vi "Write Expected Image.vi"(8 "error in (no error)":errorcluster, 10 "image data":T1, 11 "Image Assertion in":refnum<class "Image Assertion.lvclass">) -> (0 "error out":errorcluster, 3 "Image Assertion out":refnum<class "Image Assertion.lvclass">)   [LabVIEW 2020, in "MacroAssert.lvlib" / "Image Assertion.lvclass"]
uses:
  Image Assertion.lvclass
  Image Assertion.lvclass/Image Assertion.ctl
  <vilib>/picture/picture.llb/imagedata.ctl
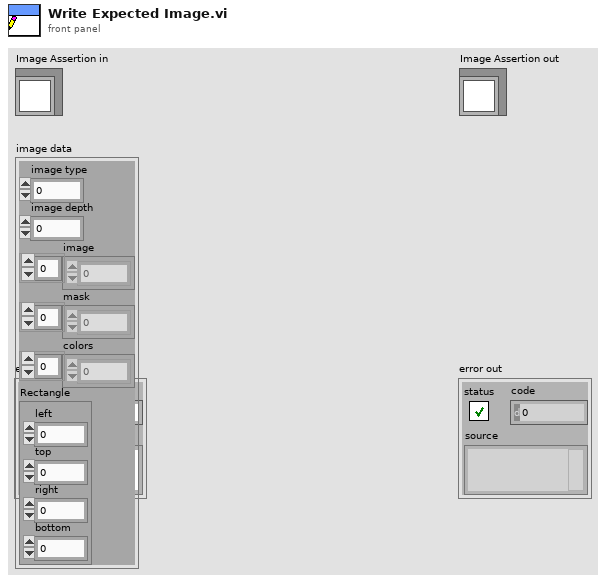
[diagram p1: front panel]
types:
  T1 = typedef "imagedata.ctl" = cluster{"image type":i32, "image depth":i32, "image":u8[], "mask":u8[], "colors":u32[], "Rectangle":cluster{"left":i16, "top":i16, "right":i16, "bottom":i16}}
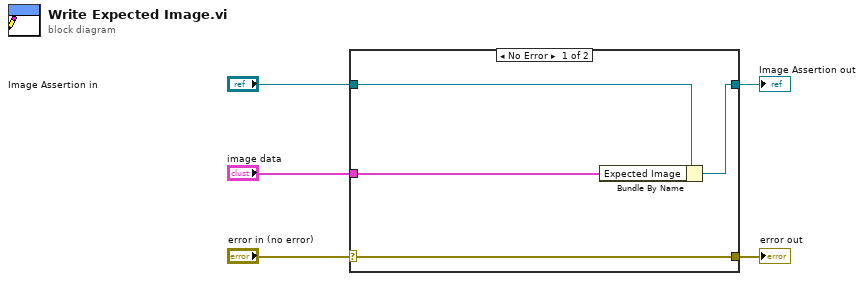
[diagram p0: block diagram]
diagram:
  n1 = case shown="No Error" "error in (no error)" {
    selector: "error in (no error)" -> [w9 w10]
    tunnel: [w9 w10] -> w4
    tunnel: [w7 w11] -> w2
    tunnel: "Image Assertion in" -> [w8 w11]
    tunnel: "image data" -> [w6 _]
    frame No Error {
      n2 = Bundle By Name(cluster=w8, "Expected Image"=w6) -> (w7:refnum<class "Image Assertion.lvclass">)
    }
    frame Error {
    }
  }
  "error out" <- w4
  "Image Assertion out" <- w2
